vi "Bus.vi"(0 "i2(k-1)":fxp<+/-,25,5>, 1 "i1(k-1)":fxp<+/-,25,5>, 2 "vo_2":fxp<+,28,8>, 3 "f1":bool, 5 "i3(k-1)":fxp<+/-,25,5>, 6 "f2":bool, 7 "vo_3":fxp<+,28,8>, 9 "T/(e*C)":fxp<+,20,0>, 11 "f3":bool, 12 "vB(k-1)":fxp<+,28,8>, 13 "vo_1":fxp<+,28,8>, 14 "1-T(R*e*C)":fxp<+,20,0>) -> (4 "vB":fxp<+,28,8>)   [LabVIEW 2015]
uses:
  <vilib>/rvi/FXPMathLib/FxpMul/XNode/nifxpmath_Multiplier.xnode
  <vilib>/rvi/FXPMathLib/FxpAdd/XNode/nifxpmath_Add.xnode
  <vilib>/rvi/FXPMathLib/sim/FxpSim.dll
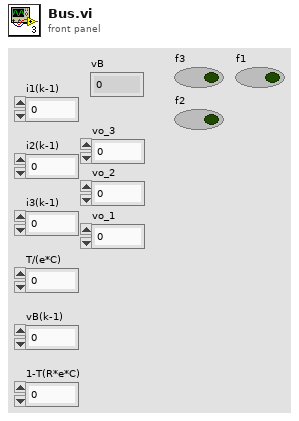
[diagram p1: front panel]
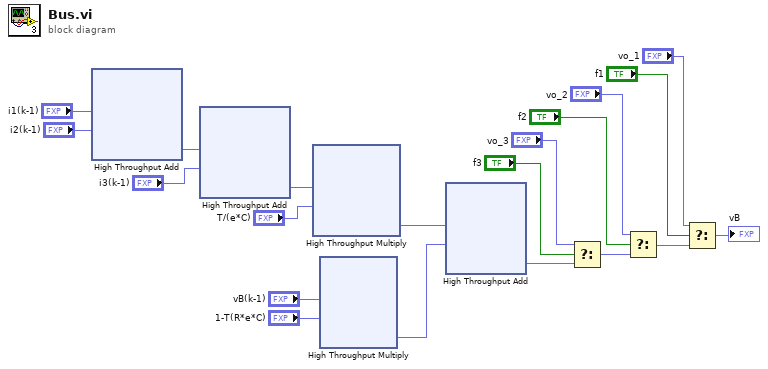
[diagram p0: block diagram]
diagram:
  n1 = xnode "High Throughput Add"("x"="i1(k-1)", "y"="i2(k-1)") -> ("x+y"=w11:fxp<+/-,26,6>)
  n2 = xnode "High Throughput Add"("x"=w11, "y"="i3(k-1)") -> ("x+y"=w15:fxp<+/-,27,7>)
  n3 = xnode "High Throughput Multiply"("x"=w15, "y"="T/(e*C)") -> ("x*y"=w17:fxp<+/-,47,7>)
  n4 = xnode "High Throughput Multiply"("x"="vB(k-1)", "y"="1-T(R*e*C)") -> ("x*y"=w18:fxp<+,48,8>)
  n5 = xnode "High Throughput Add"("x"=w17, "y"=w18) -> ("x+y"=w8:fxp<+,28,8>)
  n6 = Select(t="vo_3", s="f3", f=w8) -> (s? t:f=w9:fxp<+,28,8>)
  n7 = Select(t="vo_2", s="f2", f=w9) -> (s? t:f=w10:fxp<+,28,8>)
  n8 = Select(t="vo_1", s="f1", f=w10) -> (s? t:f=→"vB":fxp<+,28,8>)
